vi "9.5.-SubVI Identificación de Figura.vi"(10 "Array":dbl[](array[numeric]), 11 "Array 2":dbl[](array[numeric])) -> (2 "Boolean":bool, 3 "True/False":bool)   [LabVIEW 2020]
uses:
  <vilib>/Analysis/2dsp.llb/1D Cross Correlation (DBL).vi
  <vilib>/Analysis/2dsp.llb/1D Auto Correlation (DBL).vi
  <vilib>/Analysis/NI_AALPro.lvlib
panel:
  # "Visión Artificial - Firma de Figuras\nDiego Cervantes Rodríguez\ndicer0.com"
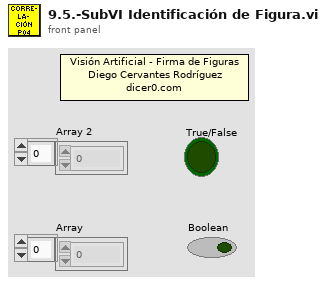
[diagram p1: front panel]
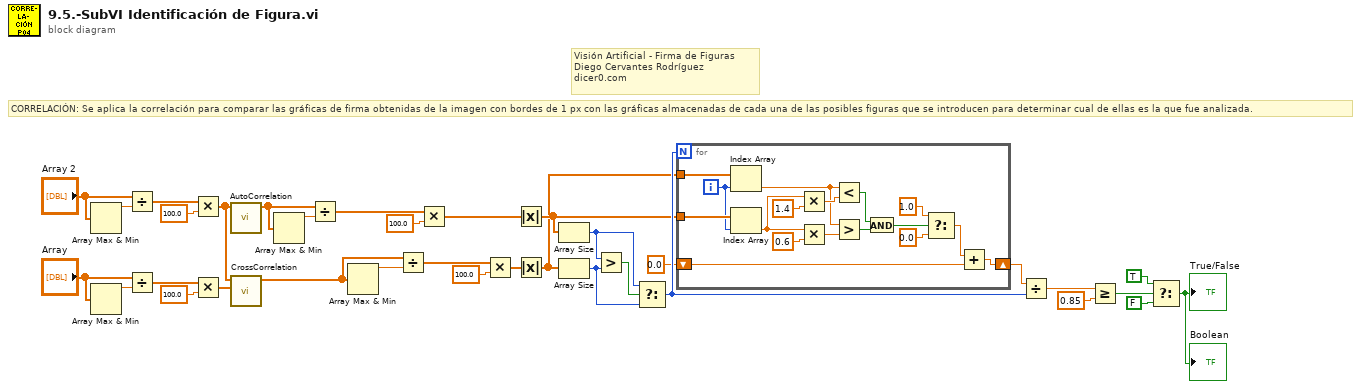
[diagram p0: block diagram]
diagram:
  # "Visión Artificial - Firma de Figuras\nDiego Cervantes Rodríguez\ndicer0.com"
  # "CORRELACIÓN: Se aplica la correlación para comparar las gráficas de firma obtenidas de la imagen con bordes de 1 px con las gráficas almacenadas de cada una de las posibles figuras que se introducen para determinar cual de ellas es la que fue analizada."
  n1 = Array Max & Min(array="Array 2") -> (max value=w1:dbl)  [unwired: 3 out]
  n2 = Array Max & Min(array="Array") -> (max value=w6:dbl)  [unwired: 3 out]
  n3 = Divide(x="Array 2", y=w1) -> (x/y=w2:dbl[])
  n4 = Divide(x="Array", y=w6) -> (x/y=w5:dbl[])
  n5 = Multiply(x=w2, y=100.0) -> (x*y=w17:dbl[])
  n6 = Multiply(x=w5, y=100.0) -> (x*y=w16:dbl[])
  n7 = call-poly <vilib>:"AutoCorrelation.vi"("X"=w17) -> ("Rxx"=w14:dbl[])  [unwired: 9 in, 1 out]
  n8 = call-poly <vilib>:"CrossCorrelation.vi"("Y"=w16, "X"=w17) -> ("Rxy"=w10:dbl[])  [unwired: 8 in, 1 out]
  n9 = Array Max & Min(array=w14) -> (max value=w13:dbl)  [unwired: 3 out]
  n10 = Divide(x=w14, y=w13) -> (x/y=w12:dbl[])
  n11 = Array Max & Min(array=w10) -> (max value=w7:dbl)  [unwired: 3 out]
  n12 = Divide(x=w10, y=w7) -> (x/y=w8:dbl[])
  n13 = Multiply(x=w12, y=100.0) -> (x*y=w18:dbl[])
  n14 = Multiply(x=w8, y=100.0) -> (x*y=w15:dbl[])
  n15 = Absolute Value(x=w18) -> (abs(x)=w23:dbl[])
  n16 = Absolute Value(x=w15) -> (abs(x)=w22:dbl[])
  n17 = Array Size(array=w23) -> (size(s)=w20:i32)
  n18 = Array Size(array=w22) -> (size(s)=w21:i32)
  n19 = Greater?(x=w20, y=w21) -> (0:w19:bool)
  n20 = Select(t=w20, s=w19, f=w21) -> (s? t:f=w26:i32)
  n21 = for {
    N: w26 -> [_]
    tunnel: w22 -> [w51]
    tunnel: w23 -> [w50]
    shift-right: [w35] -> w25
    shift-left: 0.0 ("y") -> [w37]
    i -> [w49]
    n22 = Index Array(array=w51, index=w49) -> (element=w44:dbl)
    n23 = Index Array(array=w50, index=w49) -> (element=w46:dbl)
    n24 = Multiply(x=w46, y=1.4) -> (x*y=w47:dbl)
    n25 = Multiply(x=w46, y=0.6) -> (x*y=w43:dbl)
    n26 = Less?(x=w44, y=w47) -> (x < y?=w42:bool)
    n27 = Greater?(x=w44, y=w43) -> (0:w41:bool)
    n28 = And(x=w42, y=w41) -> (x .and. y?=w40:bool)
    n29 = Select(t=1.0, s=w40, f=0.0) -> (s? t:f=w36:dbl)
    n30 = Add(x=w36, y=w37) -> (x+y=w35:dbl)
  }
  n31 = Divide(x=w25, y=w26) -> (x/y=w27:dbl)
  n32 = Greater Or Equal?(x=w27, y=0.85) -> (x >= y?=w29:bool)
  n33 = Select(t=TRUE, s=w29, f=FALSE) -> (s? t:f=→"True/False" →"Boolean":bool)
